vi "refresh.vi"(8 "error in":errorcluster, 10 "Engine Configuration In":refnum<class "engine configuration.lvclass">, 11 "Shared Memory editor node In":refnum<class "Shared Memory editor node.lvclass">) -> (0 "error out":errorcluster, 2 "Engine Configuration Out":refnum<class "engine configuration.lvclass">, 3 "Shared Memory editor node Out":refnum<class "Shared Memory editor node.lvclass">)   [LabVIEW 2013, in "Shared Memory editor node.lvclass"]
uses:
  Shared Memory editor node.lvclass
  <vilib>/NI/Module Execution Interface/Engine Configuration/engine configuration.lvclass
  <vilib>/NI/Configuration Framework/serializable configuration/get alias.vi
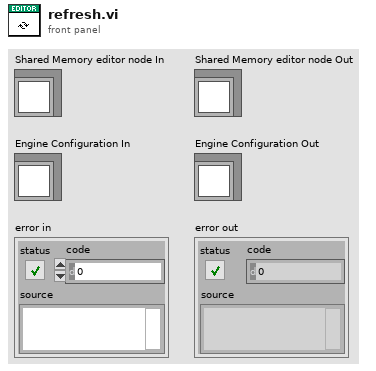
[diagram p1: front panel]
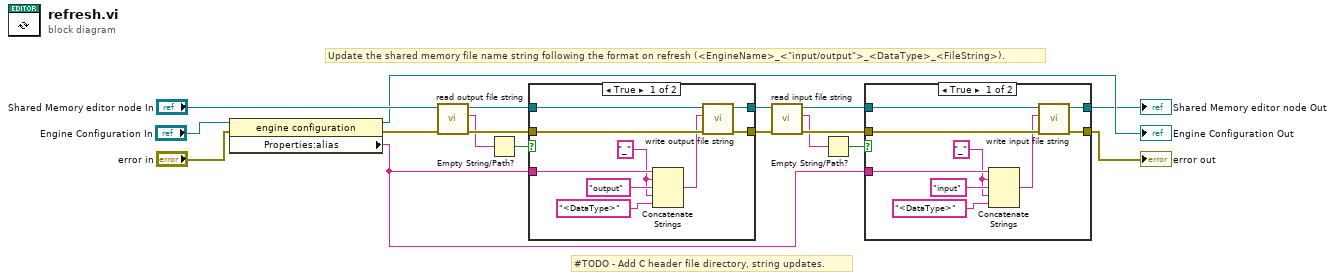
[diagram p0: block diagram]
diagram:
  # "#TODO - Add C header file directory, string updates."
  # "Update the shared memory file name string following the format on refresh (<EngineName>_<\"input/output\">_<DataType>_<FileString>)."
  n1 = property class="engine configuration"(reference="Engine Configuration In", error in="error in") -> (reference out=→"Engine Configuration Out":refnum<class "engine configuration.lvclass">, error out=w13:errorcluster, "Properties:alias"=w15:string)
  n2 = call "read output file string.vi"("error in"=w13, "shared memory editor node"="Shared Memory editor node In") -> ("error out"=w11:errorcluster, "output file string"=w2:string, "shared memory editor node out"=w12:refnum<class "Shared Memory editor node.lvclass">)  [unwired: 7 in]
  n3 = Empty String/Path?(string/path=w2) -> (empty?=w14:bool)
  n4 = case shown="True" w14 {
    tunnel: w15 -> [w23 _]
    tunnel: w12 -> [w27 w29]
    tunnel: w11 -> [w26 w28]
    tunnel: [w25 w29] -> w10
    tunnel: [w24 w28] -> w9
    frame True {
      w19 = "_" ("string")
      n5 = Concatenate Strings(w23, w19, "output", w19, "<DataType>") -> (w21:string)
      n6 = call "write output file string.vi"("error in"=w26, "output file string"=w21, "shared memory editor node"=w27) -> ("error out"=w24:errorcluster, "shared memory editor node out"=w25:refnum<class "Shared Memory editor node.lvclass">)  [unwired: 7 in]
    }
    frame False {
    }
  }
  n7 = call "read input file string.vi"("error in"=w9, "shared memory editor node"=w10) -> ("error out"=w18:errorcluster, "input file string"=w1:string, "shared memory editor node out"=w17:refnum<class "Shared Memory editor node.lvclass">)  [unwired: 7 in]
  n8 = Empty String/Path?(string/path=w1) -> (empty?=w16:bool)
  n9 = case shown="True" w16 {
    tunnel: w15 -> [w34 _]
    tunnel: w17 -> [w38 w40]
    tunnel: w18 -> [w37 w39]
    tunnel: [w36 w40] -> w4
    tunnel: [w35 w39] -> w3
    frame True {
      w30 = "_" ("string")
      n10 = Concatenate Strings(w34, w30, "input", w30, "<DataType>") -> (w32:string)
      n11 = call "write input file string.vi"("error in"=w37, "input file string"=w32, "shared memory editor node"=w38) -> ("error out"=w35:errorcluster, "shared memory editor node out"=w36:refnum<class "Shared Memory editor node.lvclass">)  [unwired: 7 in]
    }
    frame False {
    }
  }
  "Shared Memory editor node Out" <- w4
  "error out" <- w3
